vi "Untitled 6.vi"() -> ()   [LabVIEW 2012]
uses:
  <vilib>/vision/Image Controls.llb/IMAQ Image.ctl
  <vilib>/vision/NI_Vision_Development_Module.lvlib
panel:
  out "Image Dst Out":T1
  out "Read String":string
  out "ROI Descriptor":T2 {"Contours"."Type" items=["No Selection", "Point", "Line", "Rectangle", "Oval", "Polygon", "Freehand Region", "Annulus", "Unused2", "Unused3", "Broken Line", "Freehand Line", "Rotated Rectangle"]}
  out "Image Out 2":T1(plugin-control)
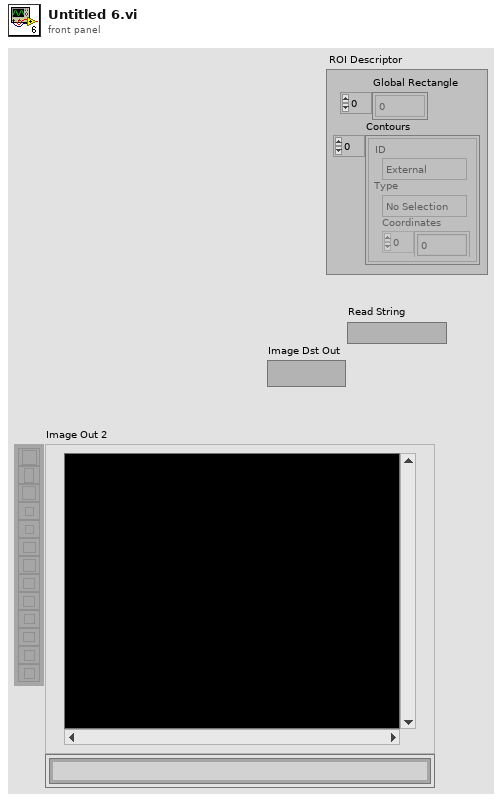
[diagram p1: front panel]
types:
  T1 = typedef "IMAQ Image.ctl" = refnum<image>
  T2 = typedef "ROI Descriptor" = cluster{"Global Rectangle":i32[], "Contours":cluster{"ID":enum32{"External", "Internal"}, "Type":u32, "Coordinates":i32[]}[]}
  T3 = typedef "IMAQ Rectangle" = cluster{"Left":i32, "Top":i32, "Right":i32, "Bottom":i32, "Rotation":dbl}
  T4 = typedef "IMAQ OCR Session.ctl" = refnum<k1>
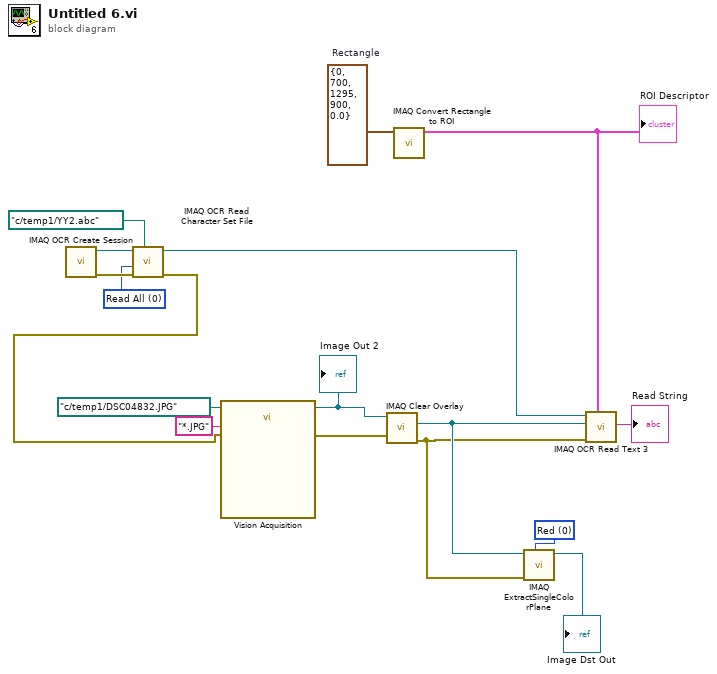
[diagram p0: block diagram]
diagram:
  w4 = 0 items=["Red", "Green", "Blue", "Hue", "Saturation", "Luminance", "Value", "Intensity"] ("Color Plane")
  w8 = T3 {"Left"=0, "Top"=700, "Right"=1295, "Bottom"=900, "Rotation"=0.0}  # Rectangle
  w11 = 0 items=["Read All", "Read Character Set Only", "Read Properties Only"] ("Read Options")
  n1 = call "IMAQ OCR Create Session"() -> ("error out"=w12:errorcluster, "IMAQ OCR Session"=w13:T4)  [unwired: 1 in, 9 out]
  n2 = call "IMAQ OCR Read Character Set File"("File Path"=path "c:/temp1/YY2.abc", "error in (no error)"=w12, "Read Options"=w11, "IMAQ OCR Session"=w13) -> ("error out"=w10:errorcluster, "IMAQ OCR Session (dup)"=w9:T4)  [unwired: 1 in, 5 out]
  n3 = call "Vision Acquisition"("Image Path"=path "c:/temp1/DSC04832.JPG", "Image File Type (All Types)"="*.JPG", "error in"=w10) -> ("Image Out"=w15:T1, "error out"=w14:errorcluster)  [unwired: 22 in, 1 out]
  "Image Out 2" <- w15
  n4 = call "IMAQ Clear Overlay"("error in (no error)"=w14, "Image"=w15) -> ("error out"=w2:errorcluster, "Image Out"=w3:T1)  [unwired: 1 in, 7 out]
  n5 = call "IMAQ Convert Rectangle to ROI"("Rectangle"=w8) -> ("ROI Descriptor"=w7:T2)  [unwired: 8 in, 1 out]
  "ROI Descriptor" <- w7
  n6 = call "IMAQ ExtractSingleColorPlane"("Color Plane"=w4, "error in (no error)"=w2, "Image Src"=w3) -> ("Image Dst Out"=→"Image Dst Out":T1)  [unwired: 7 in, 1 out]
  n7 = call "IMAQ OCR Read Text 3"("ROI Descriptor"=w7, "error in (no error)"=w2, "Image"=w3, "IMAQ OCR Session"=w9) -> ("Read String"=→"Read String":string)  [unwired: 1 in, 6 out]
